vi "Read Dynamic Data Info.vi"(7 "Unit ID (A)":string="A", 8 "error in":errorcluster, 10 "Software Rev":u8, 11 "VISA Session In":refnum<visa-resource-name>="Alicat") -> (0 "error out":errorcluster, 1 "Dynamic Data Info":T1, 3 "VISA Session Out":refnum<visa-resource-name>)   [LabVIEW 2015]
doc: "Returns the data information from firmware revision 6 units and above. The outputs are arrays containing the data variable, the data units, and whether or not the data is a string (array indexes are matched to the order that the data columns appear in the serial data frame). This VI is to be paired with the \"Read Dynamic Measurements\" VI."
uses:
  <vilib>/Instr/_visa.llb/VISA Flush IO Buffer Mask.ctl
panel:
  out "Measurement Units Intermediate\n(newer revisions)":T2={"Pressure Units"=1, "Temperature Units"=1, "Volumetric Units"=1, "Mass Units"=1, "Setpoint Units"=1, "Valve Drive Units"=1, "Total Mass Units"=1, "Total Volume Units"=1, "Time Units"=1} {"Setpoint Units" items=["Default"=0, "Unknown"=1, "SuL/m"=2, "SmL/s"=3, "SmL/m"=4, "SmL/h"=5, "SL/s"=6, "SLPM"=7, "SL/h"=8, "SCCS"=11, "SCCM"=12, "Scm3/h"=13, "Sm3/m"=14, "Sm3/h"=15, "Sm3/d"=16, "Sin3/m"=17, "SCFM"=18, "SCFH"=19, "kSCFM"=20, "NuL/m"=32, "NmL/s"=33, "NmL/m"=34, "NmL/h"=35, "NL/s"=36, "NLPM"=37, "NL/h"=38, "NCCS"=41, "NCCM"=42, "Ncm3/h"=43, "Nm3/m"=44, "Nm3/h"=45, "Nm3/d"=46, "count"=62, "%"=63, "mg/s"=64, "mg/m"=65, "g/s"=66, "g/m"=67, "g/h"=68, "kg/m"=69, "kg/h"=70, "oz/s"=71, "oz/m"=72, "lb/m"=73, "lb/h"=74]; "Time Units" items=["Default", "Unknown", "h:m:s", "ms", "s", "m", "hour", "day"]; "Total Volume Units" items=["Default"=0, "Unknown"=1, "uL"=2, "mL"=3, "L"=4, "US GAL"=5, "cm3"=6, "m3"=7, "in3"=8, "ft3"=9, "uP"=61]; "Total Mass Units" items=["Default"=0, "Unknown"=1, "SuL"=2, "SmL"=3, "SL"=4, "Scm3"=6, "Sm3"=7, "Sin3"=8, "Sft3"=9, "kSft3"=10, "NuL"=32, "NmL"=33, "NL"=34, "Ncm3"=35, "Nm3"=36, "mg"=64, "g"=65, "kg"=66, "oz"=67, "lb"=68]; "Valve Drive Units" items=["Default"=0, "Unknown"=1, "count"=2, "%"=63]; "Mass Units" items=["Default"=0, "Unknown"=1, "SuL/m"=2, "SmL/s"=3, "SmL/m"=4, "SmL/h"=5, "SL/s"=6, "SLPM"=7, "SL/h"=8, "SCCS"=11, "SCCM"=12, "Scm3/h"=13, "Sm3/m"=14, "Sm3/h"=15, "Sm3/d"=16, "Sin3/m"=17, "SCFM"=18, "SCFH"=19, "kSCFM"=20, "NuL/m"=32, "NmL/s"=33, "NmL/m"=34, "NmL/h"=35, "NL/s"=36, "NLPM"=37, "NL/h"=38, "NCCS"=41, "NCCM"=42, "Ncm3/h"=43, "Nm3/m"=44, "Nm3/h"=45, "Nm3/d"=46, "count"=62, "%"=63, "mg/s"=64, "mg/m"=65, "g/s"=66, "g/m"=67, "g/h"=68, "kg/m"=69, "kg/h"=70, "oz/s"=71, "oz/m"=72, "lb/m"=73, "lb/h"=74]; "Volumetric Units" items=["Default"=0, "Unknown"=1, "uL/m"=2, "mL/s"=3, "mL/m"=4, "mL/h"=5, "L/s"=6, "LPM"=7, "L/h"=8, "US GPM"=9, "US GPH"=10, "CCS"=11, "CCM"=12, "cm3/h"=13, "m3/m"=14, "m3/h"=15, "m3/d"=16, "in3/m"=17, "CFM"=18, "CFH"=19, "count"=62, "%"=63]; "Temperature Units" items=["Default", "Unknown", "°C", "°F", "K", "°Ra"]; "Pressure Units" items=["Default"=0, "Unknown"=1, "Pa"=2, "hPa"=3, "kPa"=4, "MPa"=5, "mbar"=6, "bar"=7, "g/cm2"=8, "kg/cm"=9, "PSI"=10, "PSF"=11, "mTorr"=12, "torr"=13, "mmHg"=14, "inHg"=15, "mmH2O"=16, "mmH2O"=17, "cmH2O"=18, "cmH2O"=19, "inH2O"=20, "inH2O"=21, "atm"=22, "m asl"=23, "ft asl"=24, "V"=61, "count"=62, "%"=63]}
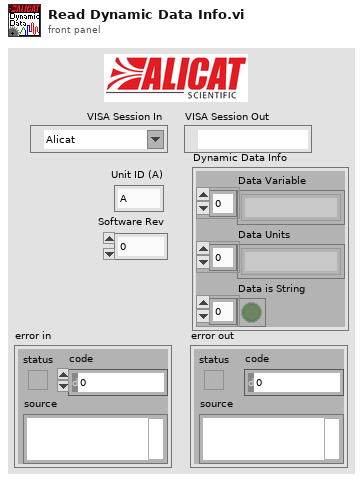
[diagram p1: front panel]
types:
  T1 = cluster{"Data Variable":string[], "Data Units":string[], "Data is String":bool[]}
  T2 = cluster{"Pressure Units":u16, "Temperature Units":u16, "Volumetric Units":u16, "Mass Units":u16, "Setpoint Units":u16, "Valve Drive Units":u16, "Total Mass Units":u16, "Total Volume Units":u16, "Time Units":u16}
  T3 = typedef "VISA Flush IO Buffer Mask.ctl" = u16
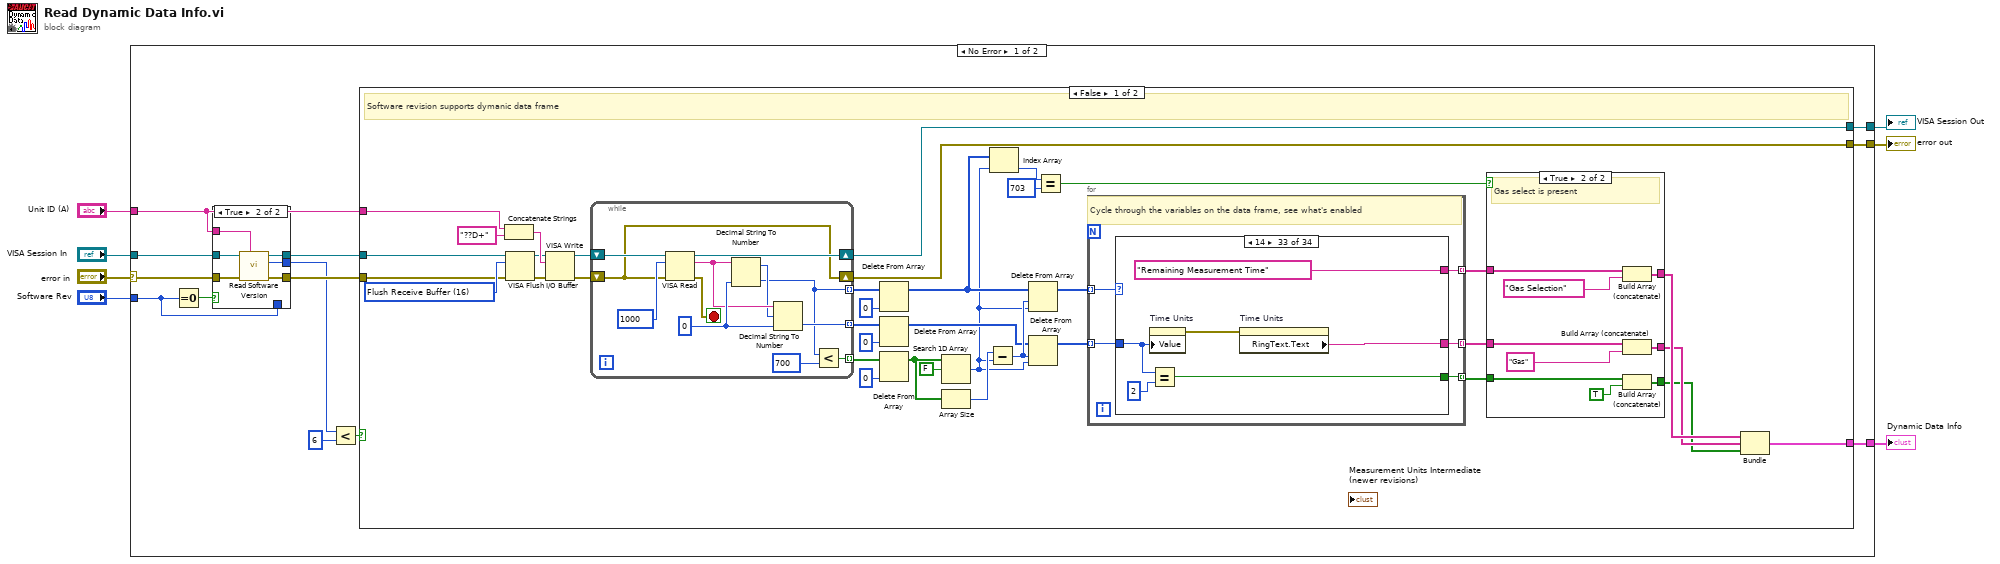
[diagram p0: block diagram]
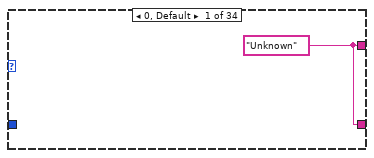
[diagram p4: hidden frame]
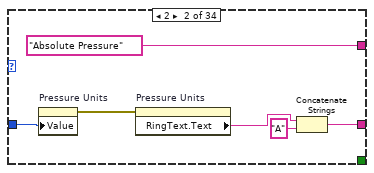
[diagram p5: hidden frame]
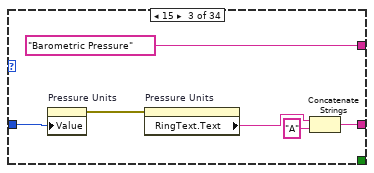
[diagram p6: hidden frame]
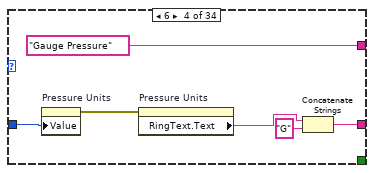
[diagram p7: hidden frame]
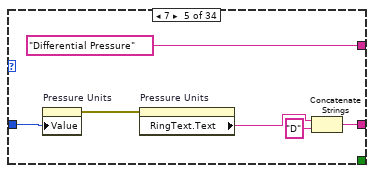
[diagram p8: hidden frame]
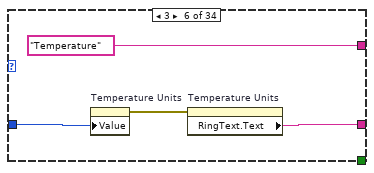
[diagram p9: hidden frame]
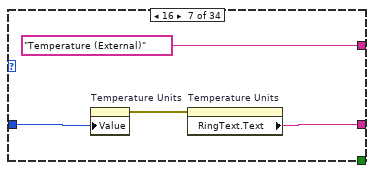
[diagram p10: hidden frame]
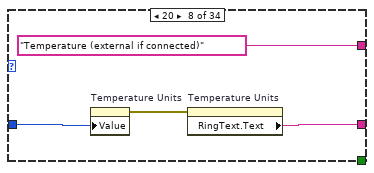
[diagram p11: hidden frame]
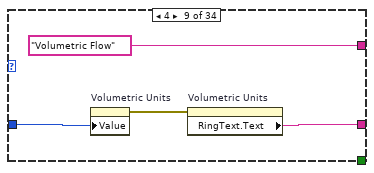
[diagram p12: hidden frame]
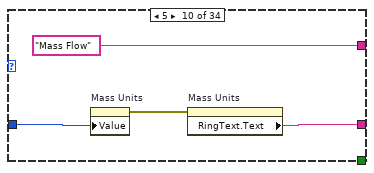
[diagram p13: hidden frame]
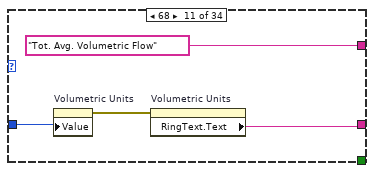
[diagram p14: hidden frame]
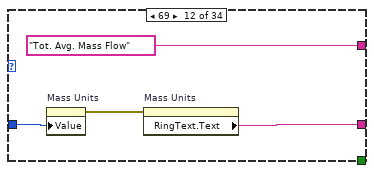
[diagram p15: hidden frame]
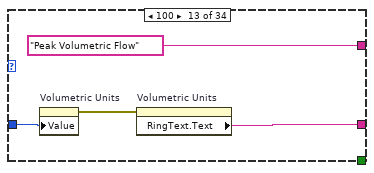
[diagram p16: hidden frame]
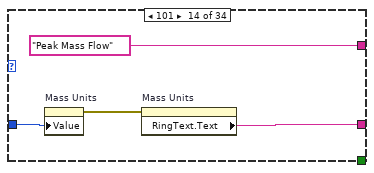
[diagram p17: hidden frame]
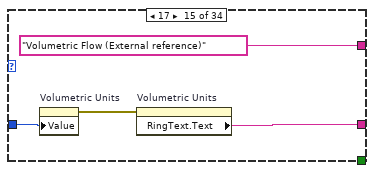
[diagram p18: hidden frame]
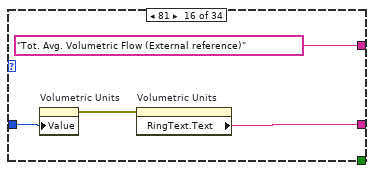
[diagram p19: hidden frame]
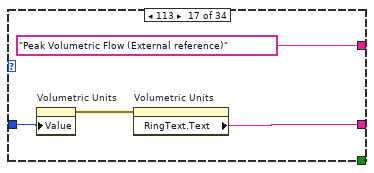
[diagram p20: hidden frame]
diagram:
  n1 = case shown="No Error" "error in" {
    selector: "error in" -> [w8 w249]
    tunnel: [w18 w248] -> w7
    tunnel: "VISA Session In" -> [w15 w248]
    tunnel: "Unit ID (A)" -> [w13 _]
    tunnel: "Software Rev" -> [w12 _]
    tunnel: [w10 cluster{string[], string[], bool[]} {[], [], []}] -> w3
    tunnel: [w9 w249] -> w2
    frame No Error {
      n2 = Equal To 0?(x=w12) -> (x = 0?=w17:bool)
      n3 = case shown="True" w17 {
        tunnel: w8 -> [w22 w29]
        tunnel: w15 -> [w21 w28]
        tunnel: w13 -> [_ w27]
        tunnel: [w22 w26] -> w16
        tunnel: [w21 w25] -> w14
        tunnel: [w23 w24] -> w11
        tunnel: w12 -> [w23 _]
        frame False {
        }
        frame True {
          n4 = call "Read Software Version.vi"("Unit ID (A)"=w27, "error in"=w29, "VISA Session In"=w28) -> ("error out"=w26:errorcluster, "Software Version"=w24:u8, "VISA Session Out"=w25:refnum<visa-resource-name>)  [unwired: 6 in]
        }
      }
      n5 = Less?(x=w11, y=u8 6) -> (x < y?=w19:bool)
      n6 = case shown="False" w19 {
        tunnel: w16 -> [w59 w246]
        tunnel: w14 -> [w58 w245]
        tunnel: w13 -> [w57 _]
        tunnel: [w35 w246] -> w9
        tunnel: [w34 w245] -> w18
        tunnel: [w30 cluster{string[], string[], bool[]} {[], [], []}] -> w10
        frame False {
          w62 = T3 16 items=["Flush Receive Buffer"=16, "Write Transmit Buffer to Device"=32, "Flush Receive Buffer (No I/O)"=64, "Flush Transmit Buffer"=128] ("Mask")
          # "Software revision supports dymanic data frame"
          n7 = Concatenate Strings(w57, "??D+" ("string")) -> (w66:string)
          n8 = VISA Flush I/O Buffer(VISA resource name=w58, mask (16)=w62, error in (no error)=w59) -> (VISA resource name out=w63:refnum<visa-resource-name>, error out=w64:errorcluster)
          n9 = VISA Write(VISA resource name=w63, write buffer=w66, error in (no error)=w64) -> (VISA resource name out=w44:refnum<visa-resource-name>, error out=w45:errorcluster)  [unwired: 1 out]
          n10 = while {
            shift-right: [w88] -> w34
            shift-left: w44 -> [w89]
            shift-right: [w87] -> w35
            shift-left: w45 -> [w87]
            tunnel: [w86] -> w53 mode=indexing
            tunnel: [w79] -> w52 mode=indexing
            tunnel: [w80] -> w48 mode=indexing
            stop <- w85 stop-if-true
            w83 = u16 0 ("default value 2")
            n11 = VISA Read(VISA resource name=w89, byte count=u32 1000, error in (no error)=w87) -> (VISA resource name out=w88:refnum<visa-resource-name>, read buffer=w82:string, error out=w85:errorcluster)  [unwired: 1 out]
            n12 = Decimal String To Number(string=w82, default (0L)=w83) -> (offset past number=w81:i32, number=w79:u16)  [unwired: 1 in]
            n13 = Decimal String To Number(string=w82, offset=w81, default (0L)=w83) -> (number=w80:u16)  [unwired: 1 out]
            n14 = Less?(x=w79, y=u16 700) -> (x < y?=w86:bool)
          }
          n15 = Delete From Array(array=w52, index=0) -> (array with subset deleted=w42:u16[])  [unwired: 1 in, 1 out]
          n16 = Delete From Array(array=w48, index=0) -> (array with subset deleted=w46:u16[])  [unwired: 1 in, 1 out]
          n17 = Delete From Array(array=w53, index=0) -> (array with subset deleted=w51:bool[])  [unwired: 1 in, 1 out]
          n18 = Search 1D Array(1D array=w51, element=FALSE) -> (index of element=w41:i32)  [unwired: 1 in]
          n19 = Array Size(array=w51) -> (size(s)=w55:i32)
          n20 = Subtract(x=w55, y=w41) -> (x-y=w47:i32)
          n21 = Index Array(array=w42, index=w41) -> (element=w61:u16)
          n22 = Delete From Array(array=w42, length=w47, index=w41) -> (array with subset deleted=w43:u16[])  [unwired: 1 out]
          n23 = Delete From Array(array=w46, length=w47, index=w41) -> (array with subset deleted=w40:u16[])  [unwired: 1 out]
          n24 = Equal?(x=w61, y=u16 703) -> (x = y?=w39:bool)
          n25 = for {
            tunnel: w43 -> [w95] mode=indexing
            tunnel: w40 -> [w94] mode=indexing
            tunnel: [w93] -> w38 mode=indexing
            tunnel: [w92] -> w37 mode=indexing
            tunnel: [w91] -> w36 mode=indexing
            # "Cycle through the variables on the data frame, see what's enabled"
            n26 = case shown="14" w95 {
              tunnel: w94 -> [_ w100 w103 w112 w115 w122 w125 w129 w133 w137 w142 w145 w150 w154 w158 w162 w166 _ w172 w178 w184 w190 w194 w198 w202 w207 w212 w216 w220 w224 w228 w232 w236 _]
              tunnel: [w96 "Absolute Pressure" "Barometric Pressure" "Gauge Pressure" "Differential Pressure" "Temperature" "Temperature (External)" "Temperature (external if connected)" "Volumetric Flow" "Mass Flow" "Tot. Avg. Volumetric Flow" "Tot. Avg. Mass Flow" "Peak Volumetric Flow" "Peak Mass Flow" "Volumetric Flow (External reference)" "Tot. Avg. Volumetric Flow (External reference)" "Peak Volumetric Flow (External reference)" "Setpoint" "Absolute Pressure Setpoint" "Gauge Pressure Setpoint" "Differential Pressure Setpoint" "Volumetric Flow Setpoint" "Volumetric Flow Setpoint (External reference)" "Mass Flow Setpoint" "Valve Drive" "Totalizing Time" "Total Volume" "Total Volume (External Reference)" "Total Mass" "Remaining Batch, Volume" "Remaining Batch, Volume (External Reference)" "Remaining Batch, Mass" "Remaining Measurement Time" "Temperature Reference Source"] -> w93
              tunnel: [w96 w97 w105 w110 w117 w121 w126 w130 w134 w138 w141 w146 w149 w153 w157 w161 w165 "Undefined" ("RingText.Text") w171 w177 w183 w189 w193 w197 w201 w208 w211 w215 w219 w223 w227 w231 w238 "Ref." ("RingText.Text")] -> w92
              tunnel: [_ _ _ _ _ _ _ _ _ _ _ _ _ _ _ _ _ _ _ _ _ _ _ _ _ w205 _ _ _ _ _ _ w235 TRUE] -> w91
              frame 0, Default {
                w96 = "Unknown"
              }
              frame 2 {
                n27 = property on="Pressure Units" class="Ring (strict)"("Value"=w100) -> (error out=w101:errorcluster)  [unwired: 2 in, 1 out]
                n28 = property on="Pressure Units" class="Ring (strict)"(error in=w101) -> ("RingText.Text"=w98:string)  [unwired: 1 in, 2 out]
                n29 = Concatenate Strings(w98, "A" ("string")) -> (w97:string)
              }
              frame 15 {
                n30 = property on="Pressure Units" class="Ring (strict)"("Value"=w103) -> (error out=w107:errorcluster)  [unwired: 2 in, 1 out]
                n31 = property on="Pressure Units" class="Ring (strict)"(error in=w107) -> ("RingText.Text"=w104:string)  [unwired: 1 in, 2 out]
                n32 = Concatenate Strings(w104, "A" ("string")) -> (w105:string)
              }
              frame 6 {
                n33 = property on="Pressure Units" class="Ring (strict)"("Value"=w112) -> (error out=w113:errorcluster)  [unwired: 2 in, 1 out]
                n34 = property on="Pressure Units" class="Ring (strict)"(error in=w113) -> ("RingText.Text"=w109:string)  [unwired: 1 in, 2 out]
                n35 = Concatenate Strings(w109, "G" ("string")) -> (w110:string)
              }
              frame 7 {
                n36 = property on="Pressure Units" class="Ring (strict)"("Value"=w115) -> (error out=w119:errorcluster)  [unwired: 2 in, 1 out]
                n37 = property on="Pressure Units" class="Ring (strict)"(error in=w119) -> ("RingText.Text"=w116:string)  [unwired: 1 in, 2 out]
                n38 = Concatenate Strings(w116, "D" ("string")) -> (w117:string)
              }
              frame 3 {
                n39 = property on="Temperature Units" class="Ring (strict)"("Value"=w122) -> (error out=w123:errorcluster)  [unwired: 2 in, 1 out]
                n40 = property on="Temperature Units" class="Ring (strict)"(error in=w123) -> ("RingText.Text"=w121:string)  [unwired: 1 in, 2 out]
              }
              frame 16 {
                n41 = property on="Temperature Units" class="Ring (strict)"("Value"=w125) -> (error out=w127:errorcluster)  [unwired: 2 in, 1 out]
                n42 = property on="Temperature Units" class="Ring (strict)"(error in=w127) -> ("RingText.Text"=w126:string)  [unwired: 1 in, 2 out]
              }
              frame 20 {
                n43 = property on="Temperature Units" class="Ring (strict)"("Value"=w129) -> (error out=w131:errorcluster)  [unwired: 2 in, 1 out]
                n44 = property on="Temperature Units" class="Ring (strict)"(error in=w131) -> ("RingText.Text"=w130:string)  [unwired: 1 in, 2 out]
              }
              frame 4 {
                n45 = property on="Volumetric Units" class="Ring (strict)"("Value"=w133) -> (error out=w135:errorcluster)  [unwired: 2 in, 1 out]
                n46 = property on="Volumetric Units" class="Ring (strict)"(error in=w135) -> ("RingText.Text"=w134:string)  [unwired: 1 in, 2 out]
              }
              frame 5 {
                n47 = property on="Mass Units" class="Ring (strict)"("Value"=w137) -> (error out=w139:errorcluster)  [unwired: 2 in, 1 out]
                n48 = property on="Mass Units" class="Ring (strict)"(error in=w139) -> ("RingText.Text"=w138:string)  [unwired: 1 in, 2 out]
              }
              frame 68 {
                n49 = property on="Volumetric Units" class="Ring (strict)"("Value"=w142) -> (error out=w143:errorcluster)  [unwired: 2 in, 1 out]
                n50 = property on="Volumetric Units" class="Ring (strict)"(error in=w143) -> ("RingText.Text"=w141:string)  [unwired: 1 in, 2 out]
              }
              frame 69 {
                n51 = property on="Mass Units" class="Ring (strict)"("Value"=w145) -> (error out=w147:errorcluster)  [unwired: 2 in, 1 out]
                n52 = property on="Mass Units" class="Ring (strict)"(error in=w147) -> ("RingText.Text"=w146:string)  [unwired: 1 in, 2 out]
              }
              frame 100 {
                n53 = property on="Volumetric Units" class="Ring (strict)"("Value"=w150) -> (error out=w151:errorcluster)  [unwired: 2 in, 1 out]
                n54 = property on="Volumetric Units" class="Ring (strict)"(error in=w151) -> ("RingText.Text"=w149:string)  [unwired: 1 in, 2 out]
              }
              frame 101 {
                n55 = property on="Mass Units" class="Ring (strict)"("Value"=w154) -> (error out=w155:errorcluster)  [unwired: 2 in, 1 out]
                n56 = property on="Mass Units" class="Ring (strict)"(error in=w155) -> ("RingText.Text"=w153:string)  [unwired: 1 in, 2 out]
              }
              frame 17 {
                n57 = property on="Volumetric Units" class="Ring (strict)"("Value"=w158) -> (error out=w159:errorcluster)  [unwired: 2 in, 1 out]
                n58 = property on="Volumetric Units" class="Ring (strict)"(error in=w159) -> ("RingText.Text"=w157:string)  [unwired: 1 in, 2 out]
              }
              frame 81 {
                n59 = property on="Volumetric Units" class="Ring (strict)"("Value"=w162) -> (error out=w163:errorcluster)  [unwired: 2 in, 1 out]
                n60 = property on="Volumetric Units" class="Ring (strict)"(error in=w163) -> ("RingText.Text"=w161:string)  [unwired: 1 in, 2 out]
              }
              frame 113 {
                n61 = property on="Volumetric Units" class="Ring (strict)"("Value"=w166) -> (error out=w167:errorcluster)  [unwired: 2 in, 1 out]
                n62 = property on="Volumetric Units" class="Ring (strict)"(error in=w167) -> ("RingText.Text"=w165:string)  [unwired: 1 in, 2 out]
              }
              frame 32 {
              }
              frame 34 {
                n63 = property on="Pressure Units" class="Ring (strict)"("Value"=w172) -> (error out=w174:errorcluster)  [unwired: 2 in, 1 out]
                n64 = property on="Pressure Units" class="Ring (strict)"(error in=w174) -> ("RingText.Text"=w175:string)  [unwired: 1 in, 2 out]
                n65 = Concatenate Strings(w175, "A" ("string")) -> (w171:string)
              }
              frame 38 {
                n66 = property on="Pressure Units" class="Ring (strict)"("Value"=w178) -> (error out=w180:errorcluster)  [unwired: 2 in, 1 out]
                n67 = property on="Pressure Units" class="Ring (strict)"(error in=w180) -> ("RingText.Text"=w181:string)  [unwired: 1 in, 2 out]
                n68 = Concatenate Strings(w181, "G" ("string")) -> (w177:string)
              }
              frame 39 {
                n69 = property on="Pressure Units" class="Ring (strict)"("Value"=w184) -> (error out=w186:errorcluster)  [unwired: 2 in, 1 out]
                n70 = property on="Pressure Units" class="Ring (strict)"(error in=w186) -> ("RingText.Text"=w187:string)  [unwired: 1 in, 2 out]
                n71 = Concatenate Strings(w187, "D" ("string")) -> (w183:string)
              }
              frame 36 {
                n72 = property on="Volumetric Units" class="Ring (strict)"("Value"=w190) -> (error out=w191:errorcluster)  [unwired: 2 in, 1 out]
                n73 = property on="Volumetric Units" class="Ring (strict)"(error in=w191) -> ("RingText.Text"=w189:string)  [unwired: 1 in, 2 out]
              }
              frame 49 {
                n74 = property on="Volumetric Units" class="Ring (strict)"("Value"=w194) -> (error out=w195:errorcluster)  [unwired: 2 in, 1 out]
                n75 = property on="Volumetric Units" class="Ring (strict)"(error in=w195) -> ("RingText.Text"=w193:string)  [unwired: 1 in, 2 out]
              }
              frame 37 {
                n76 = property on="Mass Units" class="Ring (strict)"("Value"=w198) -> (error out=w199:errorcluster)  [unwired: 2 in, 1 out]
                n77 = property on="Mass Units" class="Ring (strict)"(error in=w199) -> ("RingText.Text"=w197:string)  [unwired: 1 in, 2 out]
              }
              frame 13 {
                n78 = property on="Valve Drive Units" class="Ring (strict)"("Value"=w202) -> (error out=w203:errorcluster)  [unwired: 2 in, 1 out]
                n79 = property on="Valve Drive Units" class="Ring (strict)"(error in=w203) -> ("RingText.Text"=w201:string)  [unwired: 1 in, 2 out]
              }
              frame 10 {
                n80 = property on="Time Units" class="Ring (strict)"("Value"=w207) -> (error out=w209:errorcluster)  [unwired: 2 in, 1 out]
                n81 = Equal?(x=w207, y=u16 2) -> (x = y?=w205:bool)
                n82 = property on="Time Units" class="Ring (strict)"(error in=w209) -> ("RingText.Text"=w208:string)  [unwired: 1 in, 2 out]
              }
              frame 8 {
                n83 = property on="Total Volume Units" class="Ring (strict)"("Value"=w212) -> (error out=w213:errorcluster)  [unwired: 2 in, 1 out]
                n84 = property on="Total Volume Units" class="Ring (strict)"(error in=w213) -> ("RingText.Text"=w211:string)  [unwired: 1 in, 2 out]
              }
              frame 18 {
                n85 = property on="Total Volume Units" class="Ring (strict)"("Value"=w216) -> (error out=w217:errorcluster)  [unwired: 2 in, 1 out]
                n86 = property on="Total Volume Units" class="Ring (strict)"(error in=w217) -> ("RingText.Text"=w215:string)  [unwired: 1 in, 2 out]
              }
              frame 9 {
                n87 = property on="Total Mass Units" class="Ring (strict)"("Value"=w220) -> (error out=w221:errorcluster)  [unwired: 2 in, 1 out]
                n88 = property on="Total Mass Units" class="Ring (strict)"(error in=w221) -> ("RingText.Text"=w219:string)  [unwired: 1 in, 2 out]
              }
              frame 11 {
                n89 = property on="Total Volume Units" class="Ring (strict)"("Value"=w224) -> (error out=w225:errorcluster)  [unwired: 2 in, 1 out]
                n90 = property on="Total Volume Units" class="Ring (strict)"(error in=w225) -> ("RingText.Text"=w223:string)  [unwired: 1 in, 2 out]
              }
              frame 19 {
                n91 = property on="Total Volume Units" class="Ring (strict)"("Value"=w228) -> (error out=w229:errorcluster)  [unwired: 2 in, 1 out]
                n92 = property on="Total Volume Units" class="Ring (strict)"(error in=w229) -> ("RingText.Text"=w227:string)  [unwired: 1 in, 2 out]
              }
              frame 12 {
                n93 = property on="Total Mass Units" class="Ring (strict)"("Value"=w232) -> (error out=w233:errorcluster)  [unwired: 2 in, 1 out]
                n94 = property on="Total Mass Units" class="Ring (strict)"(error in=w233) -> ("RingText.Text"=w231:string)  [unwired: 1 in, 2 out]
              }
              frame 14 {
                n95 = property on="Time Units" class="Ring (strict)"("Value"=w236) -> (error out=w239:errorcluster)  [unwired: 2 in, 1 out]
                n96 = Equal?(x=w236, y=u16 2) -> (x = y?=w235:bool)
                n97 = property on="Time Units" class="Ring (strict)"(error in=w239) -> ("RingText.Text"=w238:string)  [unwired: 1 in, 2 out]
              }
              frame 21 {
              }
            }
          }
          n98 = case shown="True" w39 {
            tunnel: w38 -> [w69 w78]
            tunnel: w37 -> [w68 w75]
            tunnel: w36 -> [w67 w74]
            tunnel: [w67 w72] -> w31
            tunnel: [w68 w71] -> w32
            tunnel: [w69 w70] -> w33
            frame False {
            }
            frame True {
              # "Gas select is present"
              n99 = Build Array (concatenate)(w78, "Gas Selection") -> (w70:string[])
              n100 = Build Array (concatenate)(w75, "Gas") -> (w71:string[])
              n101 = Build Array (concatenate)(w74, TRUE) -> (w72:bool[])
            }
          }
          n102 = Bundle(w33, w32, w31) -> (w30:cluster{string[], string[], bool[]})  [unwired: 1 in]
        }
        frame True {
          # "Software does not support dynamic data frame"
          n103 = One Button Dialog(message="Alicat firmware version does not support a dynamic data frame. Please use the static data frame sub-VI's (see the VI tree).") -> ()  [unwired: 1 in, 1 out]
        }
      }
    }
    frame Error {
    }
  }
  "VISA Session Out" <- w7
  "Dynamic Data Info" <- w3
  "error out" <- w2
